vi "Insert Custom Var.vi"(8 "error in (no error)":errorcluster, 9 "Value":string, 10 "Var Name":string, 11 "RSeries_CAM in":refnum<class "RSeries_CAM.lvclass">) -> (0 "error out":errorcluster, 2 "Success?":bool, 3 "RSeries_CAM out":refnum<class "RSeries_CAM.lvclass">)   [LabVIEW 2024, in "RSeries_CAM.lvlib" / "RSeries_CAM.lvclass"]
uses:
  RSeries_CAM.lvclass
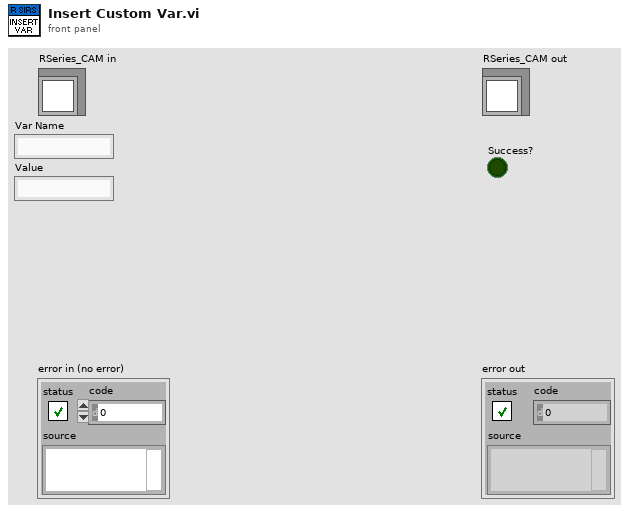
[diagram p1: front panel]
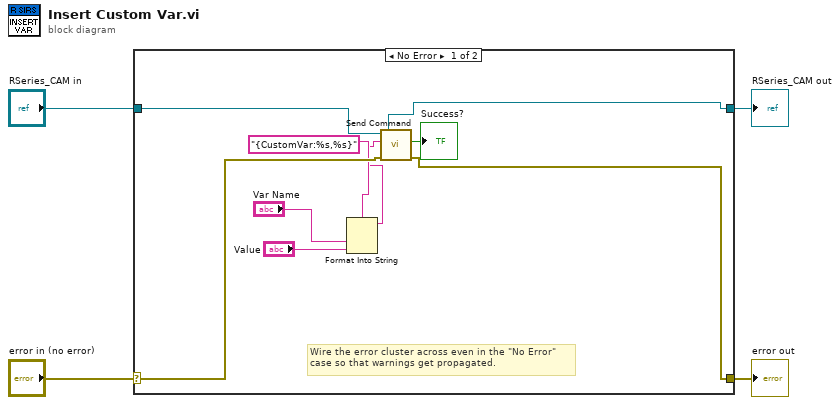
[diagram p0: block diagram]
diagram:
  n1 = case shown="No Error" "error in (no error)" {
    selector: "error in (no error)" -> [w10 w15]
    tunnel: [w9 w15] -> w3
    tunnel: [w12 w14] -> w1
    tunnel: "RSeries_CAM in" -> [w13 w14]
    frame No Error {
      # "Wire the error cluster across even in the \"No Error\"\ncase so that warnings get propagated."
      n2 = Format Into String(format string="{CustomVar:%s,%s}" ("Command"), "Var Name", "Value") -> (resulting string=w5:string)  [unwired: 2 in, 1 out]
      n3 = call "Send Command.vi"("error in (no error)"=w10, "Command"=w5, "RSeries_CAM in"=w13) -> ("error out"=w9:errorcluster, "Success?"=→"Success?":bool, "RSeries_CAM out"=w12:refnum<class "RSeries_CAM.lvclass">)  [unwired: 5 in, 1 out]
    }
    frame Error {
    }
  }
  "error out" <- w3
  "RSeries_CAM out" <- w1
